vi "KundtsTube.vi"() -> ()   [LabVIEW 2014]
panel:
  out "XY Graph":cluster{"Y":dbl[], "Y":dbl[]}[](graph)=[{"Y"=[10.0, 15.0, 20.0, 25.0, 30.0, 35.0, 40.0, 45.0, 50.0, 55.0, 60.0, 65.0, 70.0, 75.0, 80.0, 85.0, 90.0, 95.0, 100.0, 105.0, 110.0, 115.0, 120.0, 125.0, 130.0, 135.0, 140.0, 145.0, 150.0, 155.0, 160.0, 165.0, 170.0, 175.0, 180.0, 185.0, 190.0, 195.0, 200.0, 205.0, 210.0, 215.0, 220.0, 225.0, 230.0, 235.0, 240.0, 245.0, 250.0, 255.0, 260.0, 265.0, 270.0, 275.0, 280.0, 285.0, 290.0, 295.0, 300.0, 305.0, 310.0, 315.0, 320.0, 325.0, 330.0, 335.0, 340.0, 345.0, 350.0, 355.0, 360.0, 365.0, 370.0, 375.0, 380.0, 385.0, 390.0, 395.0, 400.0, 405.0, 410.0, 415.0, 420.0, 425.0, 430.0, 435.0, 440.0, 445.0, 450.0, 455.0, 460.0, 465.0, 470.0, 475.0, 480.0, 485.0, 490.0, 495.0, 500.0, 505.0, 510.0, 515.0, 520.0, 525.0, 530.0, 535.0, 540.0, 545.0, 550.0, 555.0, 560.0, 565.0, 570.0, 575.0, 580.0, 585.0, 590.0, 595.0, 600.0, 605.0, 610.0, 615.0, 620.0, 625.0, 630.0, 635.0, 640.0, 645.0, 650.0, 655.0, 660.0, 665.0, 670.0, 675.0, 680.0, 685.0, 690.0, 695.0, 700.0, 705.0, 710.0, 715.0, 720.0], "Y"=[0.005957219500424415, 0.0028576196775338407, 0.005234071949994493, 0.0052533206437485195, 0.004524812550673696, 0.00483954740948196, 0.006665275308200993, 0.007419509510364195, 0.008180960823727268, 0.009546059605990816, 0.010158490344116537, 0.011536738396282012, 0.012674734918368126, 0.013743600277114996, 0.015422702030351803, 0.0197867432932183, 0.0196175280567247, 0.02122806614139021, 0.023951345550294708, 0.02756693575880829, 0.031554334030015015, 0.035413118747998754, 0.041834268088306856, 0.04943087345648298, 0.05996101626239666, 0.07449011911325638, 0.09923598960578625, 0.13760461772897337, 0.220945205268972, 0.43102225003310707, 0.5555972226165543, 0.2954261802521254, 0.1926894088637431, 0.14215091926061513, 0.11537855899572175, 0.09959764021439911, 0.08825582077220931, 0.08010191236787169, 0.07549572697781691, 0.07107640663462862, 0.06773026466654833, 0.06574027582203289, 0.06442522089618799, 0.06373697221989974, 0.06593764509048897, 0.06461380875492101, 0.06553217973909836, 0.06747253695004232, 0.06980373481872536, 0.07280822771299045, 0.0768318119783144, 0.08165879832841996, 0.08807893924823165, 0.09579508111863197, 0.10586438755197589, 0.11862996156512087, 0.13586710014094389, 0.15920409172277314, 0.19239355244835557, 0.24333628838706325, 0.3199995618583965, 0.44417781858042005, 0.5765601464440143, 0.5408963502566124, 0.4045348797860755, 0.30437790214163407, 0.24066728586857347, 0.19999144029340354, 0.17223022970904162, 0.15307172427355928, 0.13732612938539118, 0.12625748461510677, 0.117833022460463, 0.11154368098763097, 0.10702053760666452, 0.10330559126204206, 0.10098450953661547, 0.10309868168863152, 0.09871157133438326, 0.09913872761527925, 0.09999626467544609, 0.10179940890033844, 0.10456261580906388, 0.10838747823711649, 0.11349710737714623, 0.11984621922846704, 0.12820377367881544, 0.13884845044607536, 0.15257900338670047, 0.17039790682227335, 0.19415893483883875, 0.22773202029427778, 0.27502170109944024, 0.3447283378440021, 0.4461964122235894, 0.5629884130029138, 0.5934437568933549, 0.4922550539607118, 0.37981167708272556, 0.2979067622796113, 0.24359679747628377, 0.20569182513215867, 0.17867818750665224, 0.1582445096768344, 0.1430446153993958, 0.13051870087258535, 0.12056476041393617, 0.11212770520901848, 0.10570441203384125, 0.10105671825627233, 0.09832298007407123, 0.09824739054777908, 0.09645916313598701, 0.0966956852513847, 0.09733957717107573, 0.09913292752067195, 0.10168267955993222, 0.10519974107408231, 0.1102517010146517, 0.1203234432533986, 0.12484391989996424, 0.1359004856889721, 0.15049754132589763, 0.17019574888619557, 0.19846151291573083, 0.23913592584665375, 0.3026105274965868, 0.4086754727745327, 0.5769147294974579, 0.6848389809763894, 0.535634922872796, 0.375299738562331, 0.27667304738386417, 0.2178348261299713, 0.17982135257101864, 0.1531698332734064, 0.1340216548410217, 0.12028752405156523, 0.10968989188582302, 0.10102163070486013, 0.09469374970751934, 0.08967896137253091, 0.08579503010345231]}]
  in  "Number of Samples":dbl=10000.0
  in  "Sampling Rate Hz":dbl=10000.0
  out "Waveform Graph":dynamicdata(graph)=[{"t0"=timestamp(3497988947.693461 s since 1904-01-01), "dt"=9.999999999999999e-05, "Y"=array[10000 elements], "attributes"=variant("NI_ChannelName"=variant(string "Voltage"), "NI_UnitDescription"=variant(string "Volts"))}]
  in  "Tab Control":enum32{"Sweep", "Single"}(tab)
  in  "Dwell Time (sec)":dbl=0.005
  in  "Frequency":dbl=750.0
  out "Output":cluster{"RMS":dbl, "Frequency":dbl}={"RMS"=0.08579503010345231, "Frequency"=720.0}
  in  "stop":bool
  in  "Amplitude":dbl=2.0
  in  "Sweep Settings":T1={"Minimum"=10.0, "Maximum"=10000.0, "# of Steps"=2000.0, "Spacing"=0} {"Spacing" items=["Linear", "Logarithmic"]}
  # "This will sweep from min to max, pausing by \nthe dwell time after each increment."
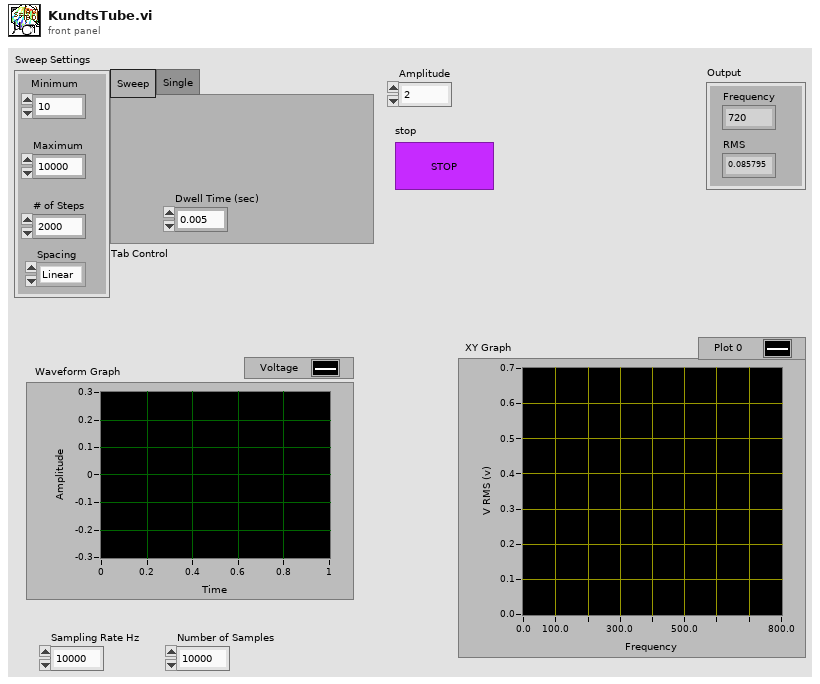
[diagram p1: front panel]
types:
  T1 = cluster{"Minimum":dbl, "Maximum":dbl, "# of Steps":dbl, "Spacing":u16}
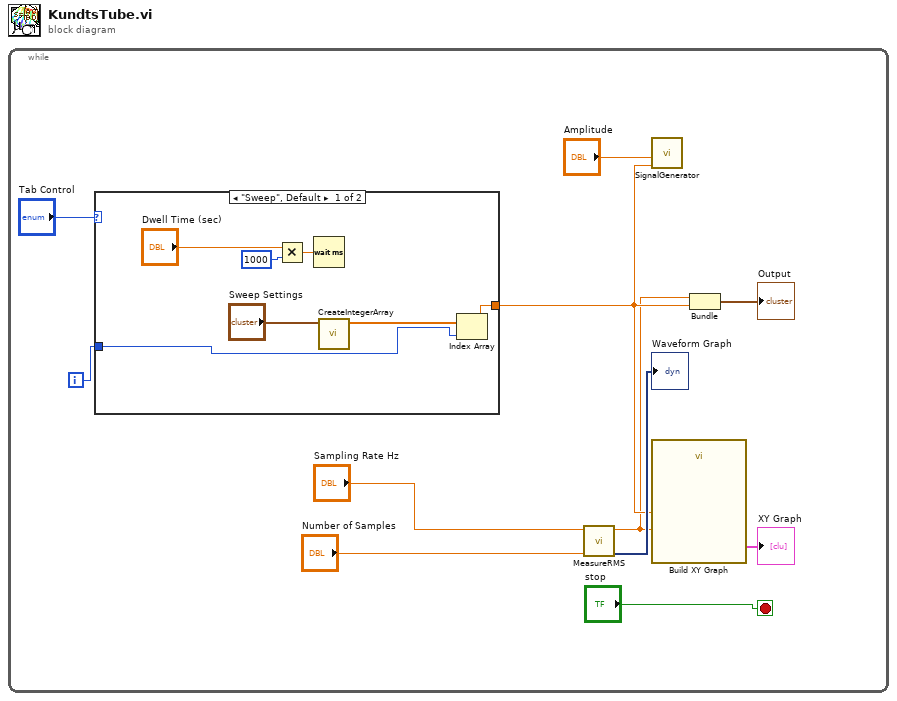
[diagram p0: block diagram]
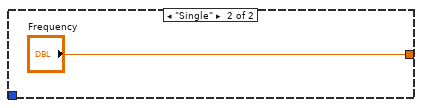
[diagram p2: hidden frame]
diagram:
  n1 = while {
    i -> [w9]
    stop <- "stop" stop-if-true
    n2 = case shown="\"Sweep\", Default" "Tab Control" {
      tunnel: w9 -> [w12 _]
      tunnel: [w13 "Frequency"] -> w5
      frame "Sweep", Default {
        n3 = Multiply(x="Dwell Time (sec)", y=1000) -> (x*y=w15:dbl)
        n4 = Wait (ms)(milliseconds to wait=w15) -> ()  [unwired: 1 out]
        n5 = call "CreateIntegerArray.vi"("Inputs"="Sweep Settings") -> ("Output Array"=w14:dbl[])  [unwired: 10 in]
        n6 = Index Array(array=w14, index=w12) -> (element=w13:dbl)
      }
      frame "Single" {
      }
    }
    n7 = call "MeasureRMS.vi"("# of Samples"="Number of Samples", "Sampling Rate (Hz)"="Sampling Rate Hz") -> ("Waveform Graph"=→"Waveform Graph":dynamicdata, "RMS"=w2:dbl)  [unwired: 8 in]
    n8 = call "SignalGenerator.vi"("Frequency"=w5, "Amplitude"="Amplitude") -> ()  [unwired: 6 in]
    n9 = call "Build XY Graph"("Y Input"=w2, "X Input"=w5) -> ("XY Graph"=→"XY Graph":cluster{"X":dbl[], "Y":dbl[]}[])  [unwired: 8 in, 1 out]
    n10 = Bundle("RMS"=w2, "Frequency"=w5) -> (→"Output":cluster{"RMS":dbl, "Frequency":dbl})  [unwired: 1 in]
  }
